vi "Page_Drivers_Read.vi"(6 "ctlReferences":T1, 8 "error in (no error)":errorcluster, 11 "Class in":refnum<class "Installer.lvclass">) -> (0 "error out":errorcluster, 3 "Class out":refnum<class "Installer.lvclass">)   [LabVIEW 2020, in "Installer.lvclass"]
uses:
  <vilib>/AppBuilder/IB_Classes/Installer/Installer.lvclass
  <vilib>/AppBuilder/IB_Classes/Installer/Installer.lvclass/Installer.ctl
  <resource>/Framework/Providers/Builds/Installer/Pages/controls/IB_UI_Page_Drivers_References.ctl
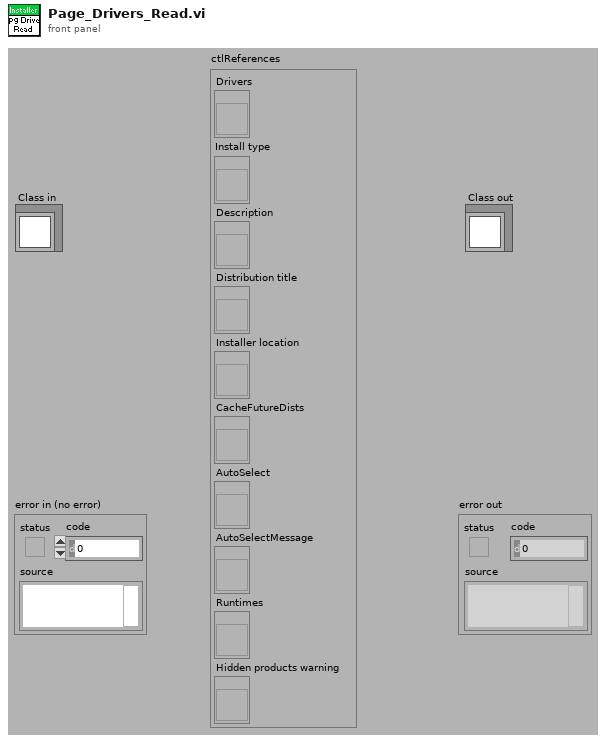
[diagram p1: front panel]
types:
  T1 = typedef "IB_UI_Page_Drivers_References.ctl" = cluster{"Drivers":refnum<vi>, "Install type":refnum<vi>, "Description":refnum<vi>, "Distribution title":refnum<vi>, "Installer location":refnum<vi>, "CacheFutureDists":refnum<vi>, "AutoSelect":refnum<vi>, "AutoSelectMessage":refnum<vi>, "Runtimes":refnum<vi>, "Hidden products warning":refnum<vi>}
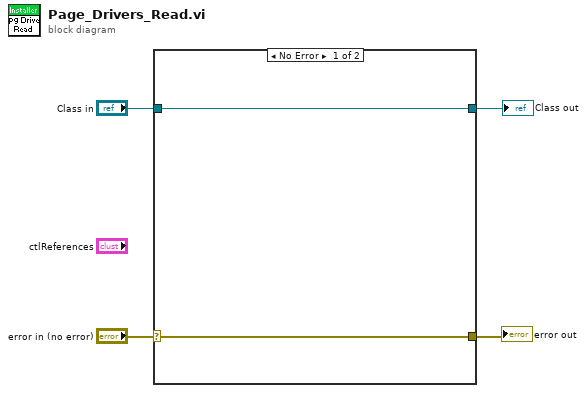
[diagram p0: block diagram]
diagram:
  n1 = case shown="No Error" "error in (no error)" {
    selector: "error in (no error)" -> [w6 w8]
    tunnel: [w6 w8] -> w3
    tunnel: [w5 w7] -> w1
    tunnel: "Class in" -> [w5 w7]
    frame No Error {
    }
    frame Error {
    }
  }
  "error out" <- w3
  "Class out" <- w1
